vi "Model.vi"() -> ()   [LabVIEW 2010]
uses:
  <vilib>/Utility/miscctls.llb/LV3DPointTypeDef.ctl
  <vilib>/picture/3D Picture Control/NI_3D Picture Control.lvlib
panel:
  in  "Z":sgl(slide)=23.292683 scale=0.0..50.0
  in  "Y":sgl(slide)=-25.609756
  out "3D Picture":refnum<vi>(3d-picture)
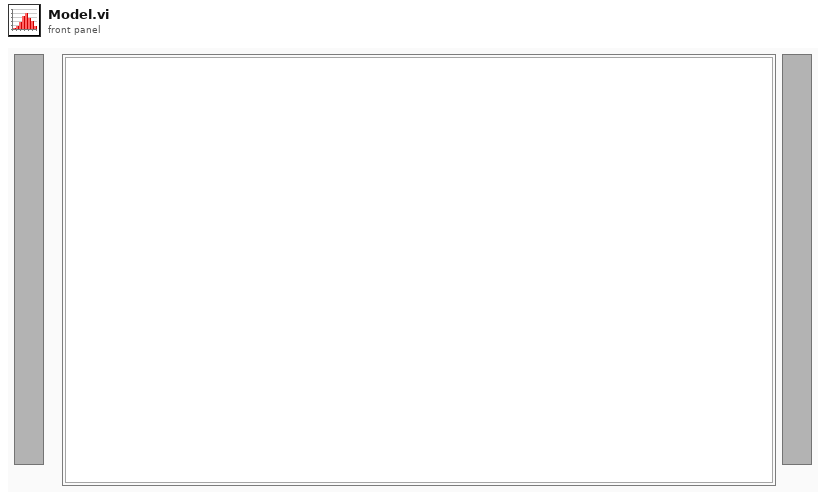
[diagram p1: front panel]
types:
  T1 = cluster{"Error":errorcluster, "PlotNames":string[], "GUIQueue":refnum<queue>, "Telemetry":string, "Format":string, "ModelRef":refnum<vi>, "Radians":dbl, "SubPanelData":string[][], "CameraAxis":dbl[]}
  T2 = typedef "LV3DPointTypeDef.ctl" = cluster{"X":sgl, "Y":sgl, "Z":sgl}
  T3 = enum32{"invalid app kind", "Development System", "Run Time System", "Student Edition", "Embedded LabVIEW", "Evaluation", "Custom"}
  T4 = cluster{"Section":string, "Key":string, "Value":string}
  T5 = cluster{"Section":string, "Key":string, "Value":string}[]
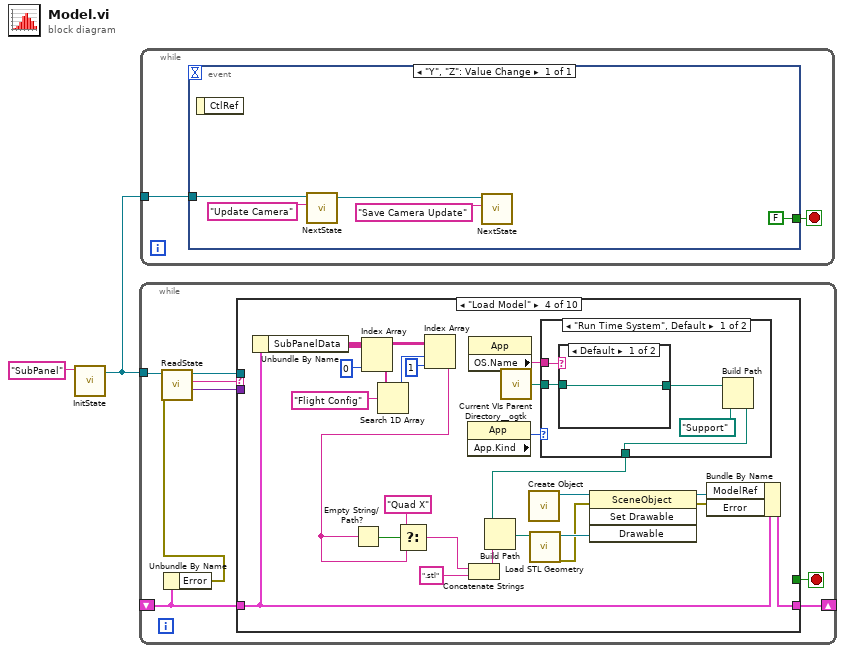
[diagram p0: block diagram]
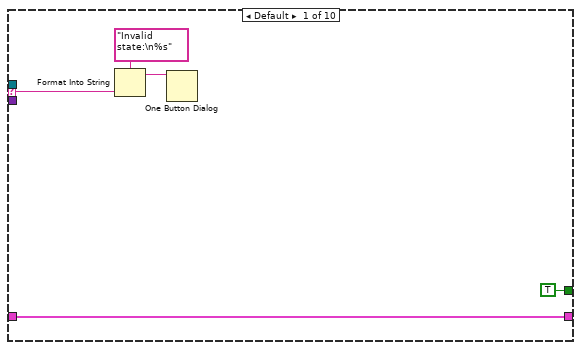
[diagram p2: hidden frame]
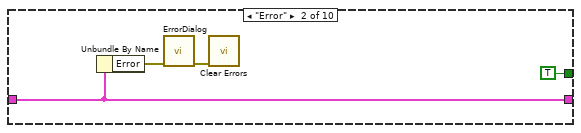
[diagram p3: hidden frame]
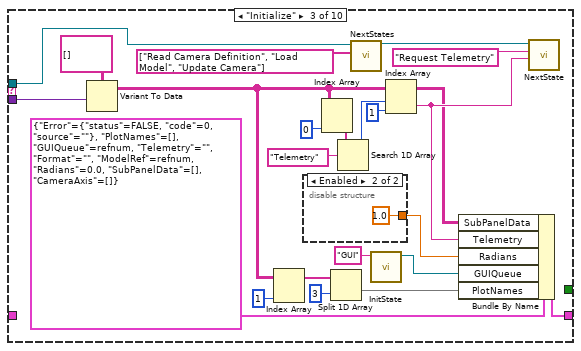
[diagram p4: hidden frame]
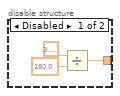
[diagram p5: hidden frame]
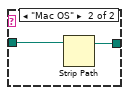
[diagram p6: hidden frame]
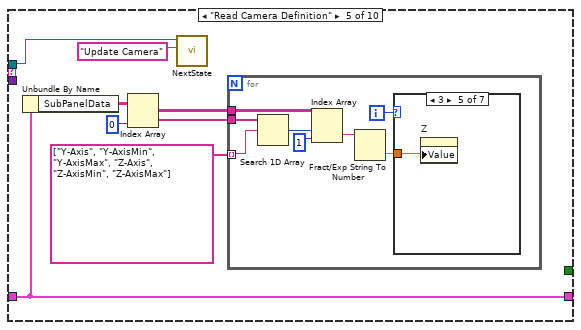
[diagram p8: hidden frame]
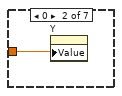
[diagram p10: hidden frame]
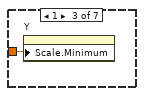
[diagram p11: hidden frame]
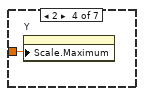
[diagram p12: hidden frame]
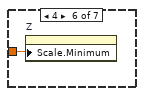
[diagram p13: hidden frame]
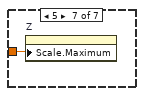
[diagram p14: hidden frame]
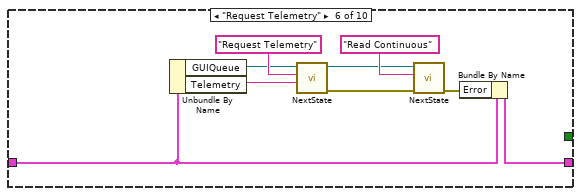
[diagram p15: hidden frame]
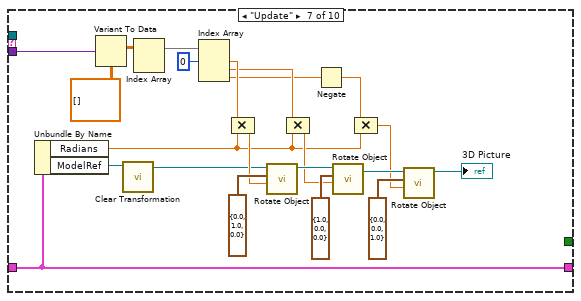
[diagram p16: hidden frame]
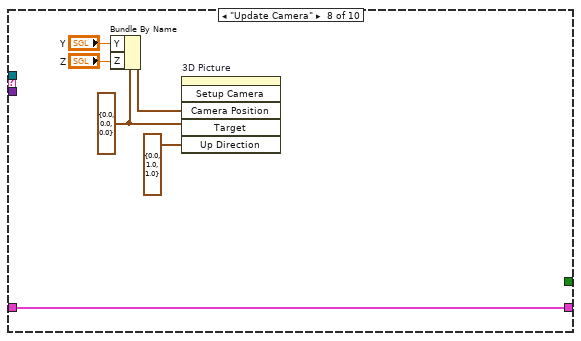
[diagram p17: hidden frame]
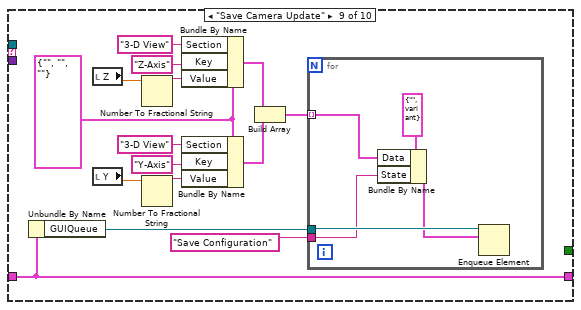
[diagram p18: hidden frame]
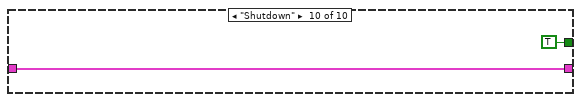
[diagram p19: hidden frame]
diagram:
  n1 = call "InitState.vi"("Name"="SubPanel" ("name (unnamed)")) -> ("Queue Out"=w1:refnum<queue>)  [unwired: 8 in, 1 out]
  n2 = while {
    tunnel: w1 -> [w7]
    shift-right: [w10] -> _
    shift-left: _ -> [w9]
    stop <- w8 stop-if-true
    n3 = Unbundle By Name(w9) -> ("Error"=w6:errorcluster)
    n4 = call "ReadState.vi"("Error In"=w6, "Queue In"=w7) -> ("Data"=w5:variant, "State"=w3:string, "Queue Out"=w4:refnum<queue>)  [unwired: 6 in, 1 out]
    n5 = case shown="\"Load Model\"" w3 {
      tunnel: w4 -> [_ _ w24 _ w80 _ _ _ _ _]
      selector: w3 -> [w13 _ _ _ _ _ _ _ _ _]
      tunnel: w5 -> [_ _ w27 _ _ _ w115 _ _ _]
      tunnel: [w12 w18 w39 w69 w81 w105 w129 w136 w137 w158] -> w10
      tunnel: w9 -> [w12 w18 _ w54 w81 w107 w129 w136 w137 w158]
      tunnel: [TRUE TRUE _ _ _ _ _ _ _ TRUE] -> w8
      frame Default {
        n6 = Format Into String(format string="Invalid state:\n%s", w13) -> (resulting string=w14:string)  [unwired: 2 in, 1 out]
        n7 = One Button Dialog(message=w14) -> ()  [unwired: 1 in, 1 out]
      }
      frame "Error" {
        n8 = Unbundle By Name(w18) -> ("Error"=w17:errorcluster)
        n9 = call "ErrorDialog.vi"("error in"=w17) -> ("error out"=w16:errorcluster)  [unwired: 10 in]
        n10 = call <vilib>:"Clear Errors.vi"("error in (no error)"=w16) -> ()  [unwired: 6 in, 1 out]
      }
      frame "Initialize" {
        n11 = Variant To Data(Variant=w27, type=string[][] [] ("subarray")) -> (data=w20:string[][])  [unwired: 1 in, 1 out]
        n12 = Index Array(array=w20, index (col)=1 ("disabled index (col)")) -> (element=w37:string[])  [unwired: 1 in]
        n13 = disable-structure shown="Enabled" {
          disable-tunnel: [w42 1.0] -> w28
          frame Disabled {
            n14 = Divide(x=3.141592653589793, y=180.0) -> (x/y=w42:dbl)
          }
          frame Enabled {
          }
        }
        n15 = Index Array(array=w20, index (col)=0 ("index (row)")) -> (element=w22:string[])  [unwired: 1 in]
        n16 = Split 1D Array(array=w37, index=3) -> (second subarray=w35:string[])  [unwired: 1 out]
        n17 = Search 1D Array(1D array=w22, element="Telemetry") -> (index of element=w30:i32)  [unwired: 1 in]
        n18 = call "NextStates.vi"("States"=string[] ["Read Camera Definition", "Load Model", "Update Camera"], "Queue In"=w24) -> ("Queue Out"=w25:refnum<queue>)  [unwired: 8 in, 1 out]
        n19 = call "InitState.vi"("Name"="GUI") -> ("Queue Out"=w33:refnum<queue>)  [unwired: 8 in, 1 out]
        n20 = Index Array(array=w20, index (row)=w30, index (col)=1 ("index (row)")) -> (element=w21:string)
        n21 = Bundle By Name(cluster=T1 {"Error"={"status"=FALSE, "code"=0, "source"=""}, "PlotNames"=[], "GUIQueue"=refnum, "Telemetry"="", "Format"="", "ModelRef"=refnum, "Radians"=0.0, "SubPanelData"=[], "CameraAxis"=[]}, "SubPanelData"=w20, "Telemetry"=w21, "Radians"=w28, "GUIQueue"=w33, "PlotNames"=w35) -> (w39:T1)
        n22 = call "NextState.vi"("Data"=w21, "State"="Request Telemetry", "Queue In"=w25) -> ()  [unwired: 7 in, 2 out]
      }
      frame "Load Model" {
        n23 = Unbundle By Name(w54) -> ("SubPanelData"=w53:string[][])
        n24 = Index Array(array=w53, index (col)=0 ("index (row)")) -> (element=w55:string[])  [unwired: 1 in]
        n25 = Search 1D Array(1D array=w55, element="Flight Config") -> (index of element=w58:i32)  [unwired: 1 in]
        n26 = Index Array(array=w53, index (row)=w58, index (col)=1 ("index (row)")) -> (element=w48:string)
        n27 = Empty String/Path?(string/path=w48) -> (empty?=w49:bool)
        n28 = Select(t="Quad X" ("string"), s=w49, f=w48) -> (s? t:f=w50:string)
        n29 = property class="App"() -> ("App.Kind"=w63:T3)  [unwired: 2 in, 2 out]
        n30 = property class="App"() -> ("OS.Name"=w60:string)  [unwired: 2 in, 2 out]
        n31 = Concatenate Strings(w50, ".stl" ("string")) -> (w52:string)
        n32 = call <userlib>:"Current VIs Parent Directory__ogtk.vi"() -> ("Parent Directory (+ Relative)"=w61:path)  [unwired: 5 in]
        n33 = call <vilib>:"Create Object.vi"() -> ("Scene:New Object"=w67:refnum<vi>)  [unwired: 2 in, 9 out]
        n34 = case shown="\"Run Time System\", Default" w63 {
          tunnel: [w74 w78] -> w62
          tunnel: w61 -> [w72 w78]
          tunnel: w60 -> [w70 _]
          frame "Run Time System", Default {
            n35 = case shown="Default" w70 {
              tunnel: [w75 w77] -> w73
              tunnel: w72 -> [w75 w76]
              frame Default {
              }
              frame "Mac OS" {
                n36 = Strip Path(path=w76) -> (stripped path=w77:path)  [unwired: 1 out]
              }
            }
            n37 = Build Path(base path=w73, name or relative path=path "Support") -> (appended path=w74:path)
          }
          frame "Development System" {
          }
        }
        n38 = Build Path(base path=w62, name or relative path=w52) -> (appended path=w46:path)
        n39 = call <vilib>:"Load STL Geometry.vi"("Model File"=w46) -> ("error out"=w66:errorcluster, "New Mesh Refnum"=w68:refnum<vi>)  [unwired: 9 in]
        n40 = invoke class="SceneObject" method="Set Drawable"(reference=w67, error in=w66, "Drawable"=w68) -> (reference out=w64:refnum<vi>, error out=w65:errorcluster)  [unwired: 1 in, 2 out]
        n41 = Bundle By Name(cluster=w54, "ModelRef"=w64, "Error"=w65) -> (w69:T1)
      }
      frame "Read Camera Definition" {
        n42 = Unbundle By Name(w81) -> ("SubPanelData"=w82:string[][])
        n43 = Index Array(array=w82, index (col)=0 ("index (row)")) -> (element=w83:string[])  [unwired: 1 in]
        n44 = call "NextState.vi"("State"="Update Camera", "Queue In"=w80) -> ()  [unwired: 8 in, 2 out]
        n45 = for {
          tunnel: string[] ["Y-Axis", "Y-AxisMin", "Y-AxisMax", "Z-Axis", "Z-AxisMin", "Z-AxisMax"] -> [w91] mode=indexing
          tunnel: w83 -> [w92]
          tunnel: w82 -> [w90]
          i -> [w87]
          n46 = Search 1D Array(1D array=w92, element=w91) -> (index of element=w93:i32)  [unwired: 1 in]
          n47 = Index Array(array=w90, index (row)=w93, index (col)=1 ("disabled index (col)")) -> (element=w88:string)
          n48 = Fract/Exp String To Number(string=w88) -> (number=w86:dbl)  [unwired: 3 in, 1 out]
          n49 = case shown="3" w87 {
            tunnel: w86 -> [_ w94 w95 w96 w97 w98 w99]
            frame Default {
            }
            frame 0 {
              n50 = property on="Y" class="Slide (strict)"("Value"=w94) -> ()  [unwired: 2 in, 2 out]
            }
            frame 1 {
              n51 = property on="Y" class="Slide (strict)"("Scale.Minimum"=w95) -> ()  [unwired: 2 in, 2 out]
            }
            frame 2 {
              n52 = property on="Y" class="Slide (strict)"("Scale.Maximum"=w96) -> ()  [unwired: 2 in, 2 out]
            }
            frame 3 {
              n53 = property on="Z" class="Slide (strict)"("Value"=w97) -> ()  [unwired: 2 in, 2 out]
            }
            frame 4 {
              n54 = property on="Z" class="Slide (strict)"("Scale.Minimum"=w98) -> ()  [unwired: 2 in, 2 out]
            }
            frame 5 {
              n55 = property on="Z" class="Slide (strict)"("Scale.Maximum"=w99) -> ()  [unwired: 2 in, 2 out]
            }
          }
        }
      }
      frame "Request Telemetry" {
        n56 = Unbundle By Name(w107) -> ("GUIQueue"=w103:refnum<queue>, "Telemetry"=w102:string)
        n57 = call "NextState.vi"("Data"=w102, "State"="Request Telemetry", "Queue In"=w103) -> ("Error Out"=w100:errorcluster, "Queue Out"=w101:refnum<queue>)  [unwired: 7 in]
        n58 = call "NextState.vi"("Error In"=w100, "State"="Read Continuous", "Queue In"=w101) -> ("Error Out"=w106:errorcluster)  [unwired: 7 in, 1 out]
        n59 = Bundle By Name(cluster=w107, "Error"=w106) -> (w105:T1)
      }
      frame "Update" {
        n60 = Unbundle By Name(w129) -> ("Radians"=w117:dbl, "ModelRef"=w128:refnum<vi>)
        n61 = Variant To Data(Variant=w115, type=dbl[][] []) -> (data=w127:dbl[][])  [unwired: 1 in, 1 out]
        n62 = call <vilib>:"Clear Transformation.vi"("Object Refnum In"=w128) -> ("Object Refnum Out"=w114:refnum<vi>)  [unwired: 9 in, 1 out]
        n63 = Index Array(array=w127) -> (element=w126:dbl[])  [unwired: 2 in]
        n64 = Index Array(array=w126, index #1=0 ("index")) -> (element #1=w121:dbl, element #2=w119:dbl, element #3=w113:dbl)  [unwired: 2 in]
        n65 = Compound Arithmetic op=MULTIPLY(w121, w117) -> (w120:dbl)
        n66 = call <vilib>:"Rotate Object.vi"("Angle"=w120, "Axis"=cluster{"X":sgl, "Y":sgl, "Z":sgl} {"X"=0.0, "Y"=1.0, "Z"=0.0}, "Scene.Object In"=w114) -> ("Scene.Object Out"=w122:refnum<vi>)  [unwired: 7 in, 1 out]
        n67 = Compound Arithmetic op=MULTIPLY(w119, w117) -> (w118:dbl)
        n68 = Negate(x=w113) -> (-x=w116:dbl)
        n69 = call <vilib>:"Rotate Object.vi"("Angle"=w118, "Axis"=cluster{"X":sgl, "Y":sgl, "Z":sgl} {"X"=1.0, "Y"=0.0, "Z"=0.0}, "Scene.Object In"=w122) -> ("Scene.Object Out"=w112:refnum<vi>)  [unwired: 7 in, 1 out]
        n70 = Compound Arithmetic op=MULTIPLY(w116, w117) -> (w109:dbl)
        n71 = call <vilib>:"Rotate Object.vi"("Angle"=w109, "Axis"=cluster{"X":sgl, "Y":sgl, "Z":sgl} {"X"=0.0, "Y"=0.0, "Z"=1.0}, "Scene.Object In"=w112) -> ("Scene.Object Out"=→"3D Picture":refnum<vi>)  [unwired: 7 in, 1 out]
      }
      frame "Update Camera" {
        w134 = T2 {"X"=0.0, "Y"=0.0, "Z"=0.0} ("Target")
        n72 = Bundle By Name(cluster=w134, "Y"="Y", "Z"="Z") -> (w133:T2)
        n73 = invoke on="3D Picture" class="SceneGraphDisp (strict)" method="Setup Camera"("Camera Position"=w133, "Target"=w134, "Up Direction"=T2 {"X"=0.0, "Y"=1.0, "Z"=1.0} ("Target")) -> ()  [unwired: 3 in, 6 out]
      }
      frame "Save Camera Update" {
        w141 = T4 {"Section"="", "Key"="", "Value"=""}
        n74 = Unbundle By Name(w137) -> ("GUIQueue"=w151:refnum<queue>)
        n75 = local read "Z"() -> (w145:sgl)
        n76 = local read "Y"() -> (w146:sgl)
        n77 = Number To Fractional String(number=w145) -> (F-format string=w144:string)  [unwired: 3 in]
        n78 = Number To Fractional String(number=w146) -> (F-format string=w147:string)  [unwired: 3 in]
        n79 = Bundle By Name(cluster=w141, "Section"="3-D View", "Key"="Z-Axis", "Value"=w144) -> (w140:T4)
        n80 = Bundle By Name(cluster=w141, "Section"="3-D View", "Key"="Y-Axis", "Value"=w147) -> (w139:T4)
        n81 = Build Array(w140, w139) -> (w138:T5)
        n82 = for {
          tunnel: w151 -> [w156]
          tunnel: "Save Configuration" ("GUI State") -> [w154]
          tunnel: w138 -> [w153] mode=indexing
          n83 = Bundle By Name(cluster=cluster{"State":string, "Data":variant} {"State"="", "Data"=variant} ("element"), "Data"=w153, "State"=w154) -> (w152:cluster{"State":string, "Data":variant})
          n84 = Enqueue Element(queue=w156, element=w152) -> ()  [unwired: 2 in, 3 out]
        }
      }
      frame "Shutdown" {
      }
    }
  }
  n85 = while {
    tunnel: w1 -> [w160]
    stop <- w159 stop-if-true
    n86 = event shown="[0] \"Y\", \"Z\": Value Change" {
      selector: _ -> [_]
      dyn-events: _ -> [_]
      timeout: _ -> [_]
      tunnel: w160 -> [w165]
      tunnel: [FALSE] -> w159
      event "Y", "Z": Value Change {
        n87 = event-data() -> ()  [unwired: 1 in, 1 out]
        n88 = call "NextState.vi"("State"="Update Camera", "Queue In"=w165) -> ("Queue Out"=w162:refnum<queue>)  [unwired: 8 in, 1 out]
        n89 = call "NextState.vi"("State"="Save Camera Update", "Queue In"=w162) -> ()  [unwired: 8 in, 2 out]
      }
    }
  }
